vi "测试循环次数.vi"() -> ()   [LabVIEW 2014]
panel:
  out "循环计数变量2":i32
  out "循环次数2":i32
  out "循环计数变量1":i32
  out "循环次数1":i32
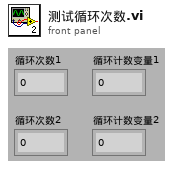
[diagram p1: front panel]
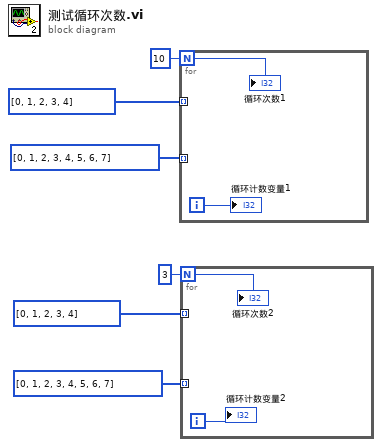
[diagram p0: block diagram]
diagram:
  n1 = for {
    N: 10 -> [w8]
    tunnel: i32[] [0, 1, 2, 3, 4] -> [_] mode=indexing
    tunnel: i32[] [0, 1, 2, 3, 4, 5, 6, 7] -> [_] mode=indexing
    i -> [w7]
    "循环次数1" <- w8
    "循环计数变量1" <- w7
  }
  n2 = for {
    N: 3 -> [w10]
    tunnel: i32[] [0, 1, 2, 3, 4, 5, 6, 7] -> [_] mode=indexing
    tunnel: i32[] [0, 1, 2, 3, 4] -> [_] mode=indexing
    i -> [w9]
    "循环次数2" <- w10
    "循环计数变量2" <- w9
  }
